vi "_AddEvent.vi"(8 "error in (no error)":errorcluster, 9 "Event":refnum<class "Event.lvclass">, 11 "EventManager in":refnum<class "EventManager.lvclass">) -> (0 "error out":errorcluster, 3 "EventManager out":refnum<class "EventManager.lvclass">)   [LabVIEW 2009, in "EventManagerLibrary.lvlib" / "EventManager.lvclass"]
uses:
  EventManager.lvclass
  EventObject/Event.lvclass
  EventManager.lvclass/EventManager.ctl
  EventBag/EventBag.lvclass
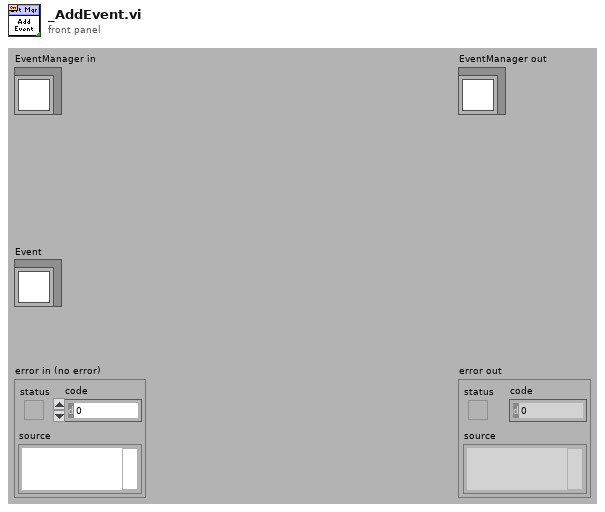
[diagram p1: front panel]
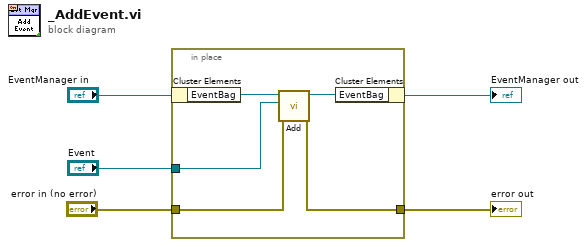
[diagram p0: block diagram]
diagram:
  n1 = in-place {
    in-place-border: "Event" -> [w6]
    in-place-border: "error in (no error)" -> [w9]
    in-place-border: [w8] -> w4
    n2 = in-place-cluster #1("EventManager in") -> ("EventBag"=w10:refnum<class "EventBag.lvclass">)
    n3 = call "Add.vi"("error in (no error)"=w9, "Event Object"=w6, "EventBag in"=w10) -> ("error out"=w8:errorcluster, "EventBag out"=w7:refnum<class "EventBag.lvclass">)  [unwired: 1 in, 6 out]
    n4 = in-place-cluster #1("EventBag"=w7) -> (→"EventManager out":refnum<class "EventManager.lvclass">)
  }
  "error out" <- w4
